vi "PXIdetect.vi"(8 "error in (no error)":errorcluster, 11 "Target (localhost)":refnum<k21>="NI-PXIe8840QuadCore-2F266B1C (192.168.150.6)") -> (0 "error out":errorcluster, 3 "PXI Available":bool)   [LabVIEW 2019]
uses:
  <vilib>/nisyscfg/Filter Mode.ctl
  <vilib>/nisyscfg/Close (Hardware).vi
  <vilib>/nisyscfg/Close (Filter).vi
  <vilib>/nisyscfg/Close (System).vi
  <vilib>/nisyscfg/nisyscfg.lvlib
  <resource>/objmgr/nisysapi.rc
  <resource>/objmgr/nicontrollersysapi.rc
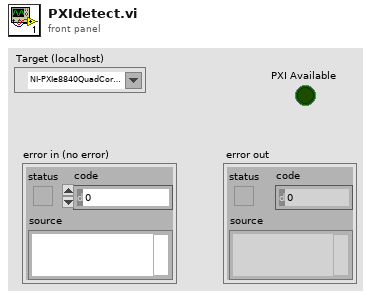
[diagram p1: front panel]
types:
  T1 = typedef "nisyscfg.lvlib/Filter Mode.ctl" = i32
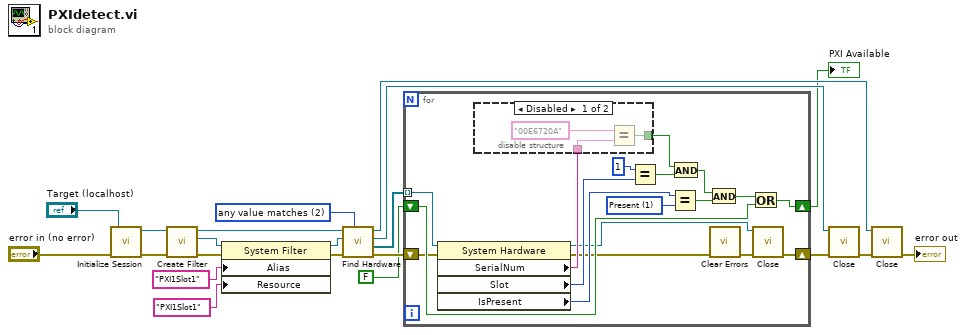
[diagram p0: block diagram]
diagram:
  w15 = T1 2 items=["all values match"=1, "any value matches"=2, "values do not match"=3, "all properties exist"=4] ("filter mode (all values match)")
  n1 = call <vilib>:"Initialize Session.vi"("error in (no error)"="error in (no error)", "Target (localhost)"="Target (localhost)") -> ("error out"=w21:errorcluster, "Session out"=w19:refnum<k21>)  [unwired: 8 in]
  n2 = call <vilib>:"Create Filter.vi"("error in (no error)"=w21, "Session in"=w19) -> ("error out"=w13:errorcluster, "Filter out"=w18:refnum<k20>, "Session out"=w17:refnum<k21>)  [unwired: 7 in]
  n3 = property class="System Filter"(reference=w18, error in=w13, "Alias"="PXI1Slot1" ("Expert Info:User Alias"), "Resource"="PXI1Slot1" ("Expert Info:Resource Name")) -> (reference out=w16:refnum<k20>, error out=w12:errorcluster)
  n4 = call <vilib>:"Find Hardware.vi"("Filter Mode (all values match)"=w15, "error in (no error)"=w12, "Filter in"=w16, "Session in"=w17) -> ("error out"=w9:errorcluster, "Resources out"=w14:refnum<k20>[], "Filter out"=w11:refnum<k20>, "Session out"=w10:refnum<k21>)  [unwired: 4 out]
  n5 = for {
    shift-right: [w29] -> w6
    shift-left: FALSE -> [w28]
    tunnel: w14 -> [w23] mode=indexing
    shift-right: [w22] -> w8
    shift-left: w9 -> [w25]
    w39 = 1 items=["Unknown"=-1, "Not Present"=0, "Present"=1] ("Devices & Chassis:Is Present")
    n6 = property class="System Hardware"(reference=w23, error in=w25) -> (reference out=w26:refnum<k20>, error out=w24:errorcluster, "SerialNum"=w35:string, "Slot"=w37:i32, "IsPresent"=w38:i32)
    n7 = disable-structure shown="Disabled" {
      disable-tunnel: w35 -> [w42 _]
      disable-tunnel: [w40 _] -> w34
      frame Disabled {
        n8 = Equal?(x="00E6720A", y=w42) -> (x = y?=w40:bool)
      }
      frame Enabled {
      }
    }
    n9 = Equal?(x=1, y=w37) -> (x = y?=w33:bool)
    n10 = Equal?(x=w38, y=w39) -> (x = y?=w31:bool)
    n11 = And(x=w34, y=w33) -> (x .and. y?=w32:bool)
    n12 = And(x=w32, y=w31) -> (x .and. y?=w30:bool)
    n13 = call <vilib>:"Clear Errors.vi"("error in (no error)"=w24) -> ("error out"=w27:errorcluster)  [unwired: 5 in, 1 out]
    n14 = Or(x=w30, y=w28) -> (x .or. y?=w29:bool)
    n15 = call-poly <vilib>:"Close.vi"("error in (no error)"=w27, "Resource in"=w26) -> ("error out"=w22:errorcluster)  [unwired: 9 in]
  }
  "PXI Available" <- w6
  n16 = call-poly <vilib>:"Close.vi"("error in (no error)"=w8, "Filter in"=w11) -> ("error out"=w7:errorcluster)  [unwired: 9 in]
  n17 = call-poly <vilib>:"Close.vi"("error in (no error)"=w7, "Session in"=w10) -> ("error out"=→"error out":errorcluster)  [unwired: 9 in]
